vi "SSC DCPower Configure Source Adapt.vi"(0 "DCPower SSC in":T2[](array[typedef]), 5 "Voltage":T1 {"Pole-Zero Ratio" format="%#_6p"; "Compensation Frequency" format="%#_6p"; "Gain Bandwidth" format="%#_6p"}, 7 "Current":T1 {"Pole-Zero Ratio" format="%#_6p"; "Compensation Frequency" format="%#_6p"; "Gain Bandwidth" format="%#_6p"}, 11 "error in":errorcluster) -> (4 "DCPower SSC out":T2[](array[typedef]), 15 "error out":errorcluster)   [LabVIEW 2020]
doc: "This VI configures Source Adapt parameters for the channels and sets them to the Custom transient response setting."
uses:
  SSC DCPower.ctl
  SSC DCPower Source Adapt.ctl
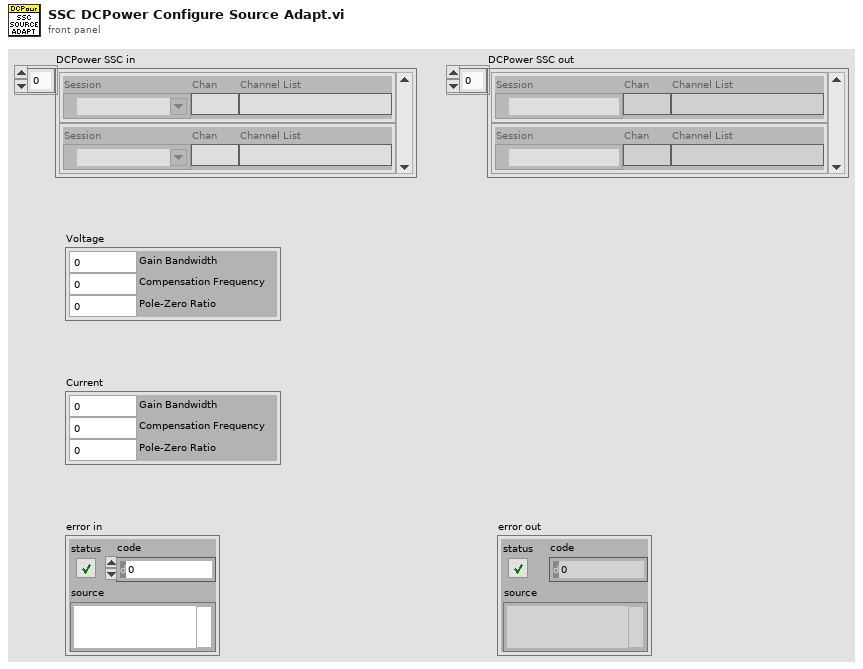
[diagram p1: front panel]
types:
  T1 = typedef "SSC DCPower Source Adapt.ctl" = cluster{"Gain Bandwidth":dbl, "Compensation Frequency":dbl, "Pole-Zero Ratio":dbl}
  T2 = typedef "SSC DCPower.ctl" = cluster{"Session":refnum<k15>, "Chan":string, "Channel List":string}
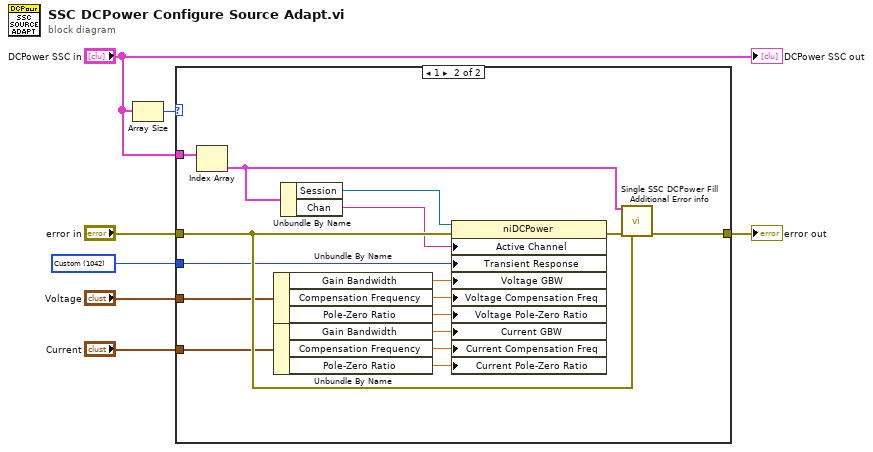
[diagram p0: block diagram]
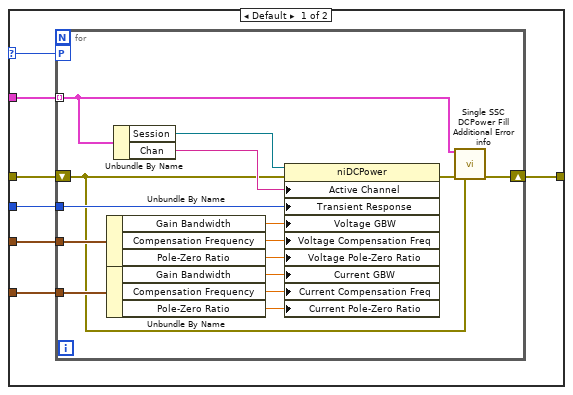
[diagram p2: hidden frame]
diagram:
  w5 = 1042 items=["Slow"=1041, "Normal"=1038, "Fast"=1039, "Custom"=1042] ("Transient Response")
  n1 = Array Size(array="DCPower SSC in") -> (size(s)=w2:i32)
  n2 = case shown="1" w2 {
    selector: w2 -> [w9 _]
    tunnel: [w14 w45] -> w7
    tunnel: "error in" -> [w13 w44]
    tunnel: w5 -> [w12 w43]
    tunnel: "Voltage" -> [w11 w42]
    tunnel: "Current" -> [w10 w41]
    tunnel: "DCPower SSC in" -> [w8 w40]
    frame Default {
      n3 = for {
        tunnel: w8 -> [w16] mode=indexing
        workers-P: w9 -> [_]
        tunnel: w12 -> [w28]
        tunnel: w11 -> [w27]
        tunnel: w10 -> [w26]
        shift-right: [w17] -> w14
        shift-left: w13 -> [w15]
        n4 = Unbundle By Name(w27) -> ("Gain Bandwidth"=w23:dbl, "Compensation Frequency"=w22:dbl, "Pole-Zero Ratio"=w21:dbl)
        n5 = Unbundle By Name(w26) -> ("Gain Bandwidth"=w20:dbl, "Compensation Frequency"=w19:dbl, "Pole-Zero Ratio"=w18:dbl)
        n6 = Unbundle By Name(w16) -> ("Session"=w25:refnum<k15>, "Chan"=w24:string)
        n7 = property class="niDCPower"(reference=w25, error in=w15, "Active Channel"=w24, "Transient Response"=w28, "Voltage GBW"=w23, "Voltage Compensation Freq"=w22, "Voltage Pole-Zero Ratio"=w21, "Current GBW"=w20, "Current Compensation Freq"=w19, "Current Pole-Zero Ratio"=w18) -> (error out=w29:errorcluster)  [unwired: 1 out]
        n8 = call "Single SSC DCPower Fill Additional Error info.vi"("DCPower SSC in"=w16, "error in"=w29, "previous error in"=w15) -> ("error out"=w17:errorcluster)  [unwired: 12 in]
      }
    }
    frame 1 {
      n9 = Index Array(array=w40) -> (element=w30:T2)  [unwired: 1 in]
      n10 = Unbundle By Name(w42) -> ("Gain Bandwidth"=w36:dbl, "Compensation Frequency"=w35:dbl, "Pole-Zero Ratio"=w34:dbl)
      n11 = Unbundle By Name(w41) -> ("Gain Bandwidth"=w33:dbl, "Compensation Frequency"=w32:dbl, "Pole-Zero Ratio"=w31:dbl)
      n12 = Unbundle By Name(w30) -> ("Session"=w38:refnum<k15>, "Chan"=w37:string)
      n13 = property class="niDCPower"(reference=w38, error in=w44, "Active Channel"=w37, "Transient Response"=w43, "Voltage GBW"=w36, "Voltage Compensation Freq"=w35, "Voltage Pole-Zero Ratio"=w34, "Current GBW"=w33, "Current Compensation Freq"=w32, "Current Pole-Zero Ratio"=w31) -> (error out=w39:errorcluster)  [unwired: 1 out]
      n14 = call "Single SSC DCPower Fill Additional Error info.vi"("DCPower SSC in"=w30, "error in"=w39, "previous error in"=w44) -> ("error out"=w45:errorcluster)  [unwired: 12 in]
    }
  }
  "error out" <- w7
  "DCPower SSC out" <- "DCPower SSC in"
